vi "Open Project Copy.vi"(8 "error in":errorcluster, 11 "Builder in":refnum<class "Builder.lvclass">) -> (0 "error out":errorcluster, 3 "Builder out":refnum<class "Builder.lvclass">)   [LabVIEW 2019, in "Builder.lvclass"]
doc: "Copies the project blankProject_<target>.lvproj into the specified directory and returns the project reference along with the directory absolute path. <b>Target Directory</b> can be an absolute path or relative to the caller."
uses:
  Builder/Builder.lvclass
  Builder/Builder.lvclass/Builder.ctl
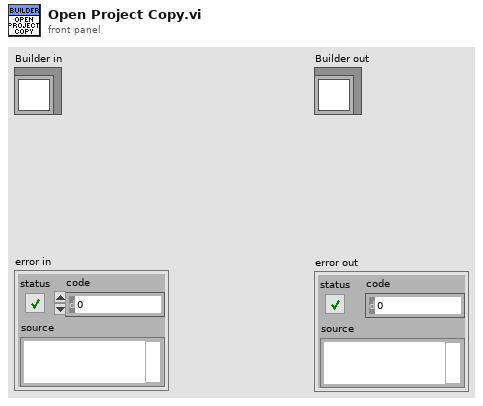
[diagram p1: front panel]
types:
  T1 = typedef "TargetType.ctl" = enum16{"Windows", "cRIO-9045"}
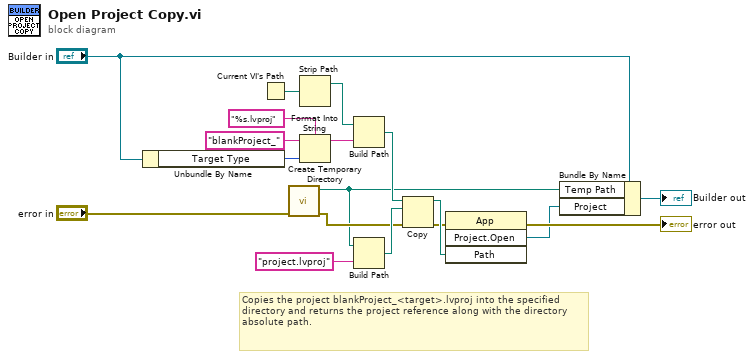
[diagram p0: block diagram]
diagram:
  # "Copies the project blankProject_<target>.lvproj into the specified directory and returns the project reference along with the directory absolute path."
  n1 = Unbundle By Name("Builder in") -> ("Target Type"=w1:T1)
  n2 = Current VI's Path() -> (path=w10:path)
  n3 = call "Create Temporary Directory.vi"("error in"="error in") -> ("error out"=w13:errorcluster, "created path"=w4:path)  [unwired: 9 in]
  n4 = Strip Path(path=w10) -> (stripped path=w14:path)  [unwired: 1 out]
  n5 = Format Into String(format string="%s.lvproj", initial string="blankProject_", w1) -> (resulting string=w11:string)  [unwired: 1 in, 1 out]
  n6 = Build Path(base path=w14, name or relative path=w11) -> (appended path=w12:path)
  n7 = Build Path(base path=w4, name or relative path="project.lvproj") -> (appended path=w15:path)
  n8 = Copy(8:w13, 10:w15, 11:w12) -> (0:w8:errorcluster, 3:w9:path)  [unwired: 2 in, 1 out]
  n9 = invoke class="App" method="Project.Open"(error in=w8, "Path"=w9) -> (error out=→"error out":errorcluster, "Project:Open"=w5:refnum<vi>)  [unwired: 2 in, 2 out]
  n10 = Bundle By Name(cluster="Builder in", "Temp Path"=w4, "Project"=w5) -> (→"Builder out":refnum<class "Builder.lvclass">)
